vi "test-PID-ALL_TESTS.vi"(8 "error in (no error)":errorcluster) -> (0 "error out":errorcluster, 3 "All Passed":bool)   [LabVIEW 2019]
panel:
  out "T3 Passed":bool
  out "T2 Passed":bool
  out "T1 Passed":bool
  out "T0 Passed":bool
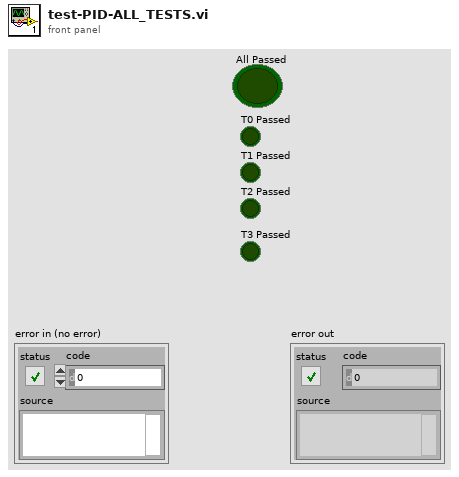
[diagram p1: front panel]
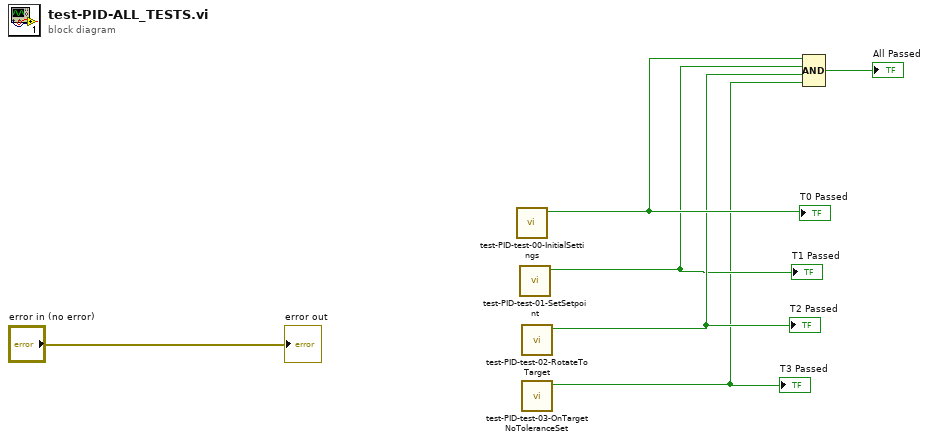
[diagram p0: block diagram]
diagram:
  n1 = call "test-PID-test-00-InitialSettings.vi"() -> ("All Passed"=w5:bool)  [unwired: 11 in]
  "T0 Passed" <- w5
  n2 = call "test-PID-test-01-SetSetpoint.vi"() -> ("All Passed"=w2:bool)  [unwired: 11 in]
  "T1 Passed" <- w2
  n3 = call "test-PID-test-02-RotateToTarget.vi"() -> ("All Passed"=w4:bool)  [unwired: 11 in]
  "T2 Passed" <- w4
  n4 = call "test-PID-test-03-OnTargetNoToleranceSet.vi"() -> ("All Passed"=w1:bool)  [unwired: 11 in]
  "T3 Passed" <- w1
  n5 = Compound Arithmetic op=AND(w5, w2, w4, w1) -> (→"All Passed":bool)
  "error out" <- "error in (no error)"
